vi "getStepNLoopParams.vi"(0 "MultiAxisController in":refnum<class "_MultiAxisController.lvclass">, 2 "axis":T2, 5 "error in (no error)":errorcluster) -> (14 "MultiAxisController out":refnum<class "_MultiAxisController.lvclass">, 16 "step_n_params":T1, 19 "error out":errorcluster)   [LabVIEW 2020, in "classes.lvlib" / "_MultiAxisController.lvclass"]
doc: "Produced By:\n\n<B>Kod Integrations, LLC</B>\n4835 Marianne Drive\nMount Airy, MD 21771\nhttp://www.kodintegrations.com\nemail: info@kodintegrations.com\nphone: (240) 687-1288"
uses:
  _MultiAxisController.lvclass
  Controller/_Controller.lvclass
  common/controls/step_n_params.ctl
  libraries/common.lvlib
  C:/GEECS/Developers Version/source/Device Drivers/Newmark-NSC-A/Arcus Driver 3.0.0/ArcusUsbComm/classes/Controller/_Controller.lvclass
  C:/GEECS/Developers Version/source/Device Drivers/Newmark-NSC-A/Arcus Driver 3.0.0/ArcusUsbComm/classes/MultiAxisController/_MultiAxisController.lvclass
  common/controls/axis.ctl
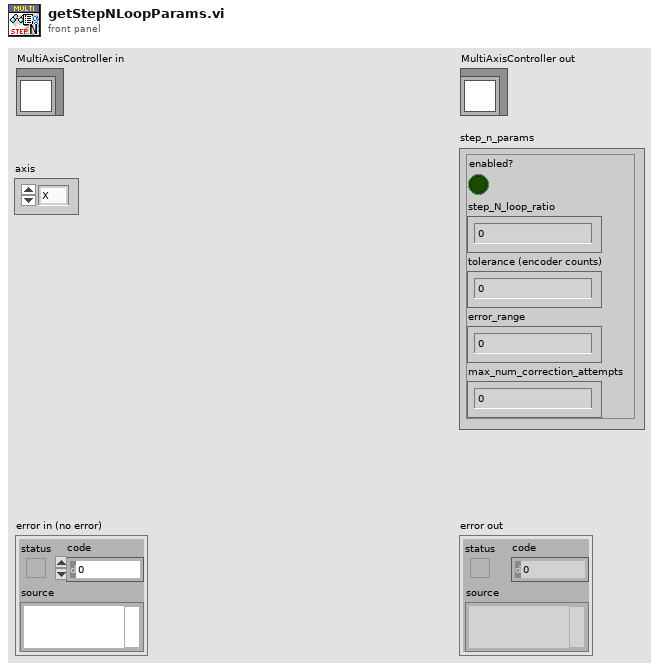
[diagram p1: front panel]
types:
  T1 = typedef "common.lvlib/step_n_params.ctl" = cluster{"step_N_loop_ratio":dbl, "tolerance (encoder counts)":u32, "error_range":i32, "max_num_correction_attempts":i32, "enabled?":bool}
  T2 = typedef "common.lvlib/axis.ctl" = enum16{"X", "Y", "Z", "U"}
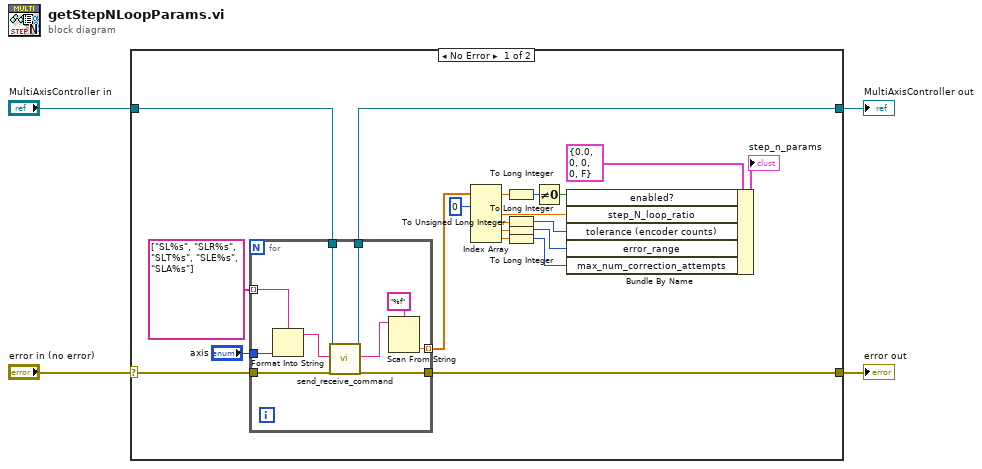
[diagram p0: block diagram]
diagram:
  n1 = case shown="No Error" "error in (no error)" {
    selector: "error in (no error)" -> [w24 w36]
    tunnel: [w23 w36] -> w3
    tunnel: [w19 w35] -> w1
    tunnel: "MultiAxisController in" -> [w20 w35]
    frame No Error {
      n2 = for {
        tunnel: w24 -> [w34]
        tunnel: [w33] -> w23
        tunnel: string[] ["SL%s", "SLR%s", "SLT%s", "SLE%s", "SLA%s"] -> [w32] mode=indexing
        tunnel: "axis" -> [w31]
        tunnel: w20 -> [w30]
        tunnel: [w29] -> w19
        tunnel: [w25] -> w17 mode=indexing
        n3 = Format Into String(format string=w32, w31) -> (resulting string=w28:string)  [unwired: 2 in, 1 out]
        n4 = call "send_receive_command.vi"("reference (in)"=w30, "ASCII Command (in)"=w28, "error in (no error)"=w34) -> ("reference (out)"=w29:refnum<class "_MultiAxisController.lvclass">, "response (out)"=w26:string, "error out"=w33:errorcluster)  [unwired: 12 in, 2 out]
        n5 = Scan From String(format string="%f", input string=w26) -> (output 1=w25:dbl)  [unwired: 3 in, 3 out]
      }
      n6 = Index Array(array=w17, index #1=0 ("index")) -> (element #1=w16:dbl, element #2=w9:dbl, element #3=w14:dbl, element #4=w12:dbl, element #5=w13:dbl)  [unwired: 4 in]
      n7 = To Long Integer(number=w16) -> (32bit integer=w15:i32)
      n8 = To Unsigned Long Integer(number=w14) -> (unsigned 32bit integer=w8:u32)
      n9 = To Long Integer(number=w12) -> (32bit integer=w7:i32)
      n10 = To Long Integer(number=w13) -> (32bit integer=w6:i32)
      n11 = Not Equal To 0?(x=w15) -> (x != 0?=w10:bool)
      n12 = Bundle By Name(cluster=T1 {"step_N_loop_ratio"=0.0, "tolerance (encoder counts)"=0, "error_range"=0, "max_num_correction_attempts"=0, "enabled?"=FALSE} ("step_n_params"), "enabled?"=w10, "step_N_loop_ratio"=w9, "tolerance (encoder counts)"=w8, "error_range"=w7, "max_num_correction_attempts"=w6) -> (→"step_n_params":T1)
    }
    frame Error {
    }
  }
  "error out" <- w3
  "MultiAxisController out" <- w1
